vi "manual.vi"() -> ()   [LabVIEW 2010]
doc: "OCW v3.0\n\nCopyright 2008 by Will Grover\n\nhttp://wgrover.com\n\nPermission is hereby granted, free of charge, to any person obtaining a copy of this software and associated documentation files (the \"Software\"), to deal in the Software without restriction, including without limitation the rights to use, copy, modify, merge, publish, distribute, sublicense, and/or sell copies of the Software, and to permit persons to whom the Software is furnished to do so, subject to the following conditions:\n\nThe above copyright notice and this permission notice shall be included in all copies or substantial portions of the Software.\n\nTHE SOFTWARE IS PROVIDED \"AS IS\", WITHOUT WARRANTY OF ANY KIND, EXPRESS OR IMPLIED, INCLUDING BUT NOT LIMITED TO THE WARRANTIES OF MERCHANTABILITY, FITNESS FOR A PARTICULAR PURPOSE AND NONINFRINGEMENT. IN NO EVENT SHALL THE AUTHORS OR COPYRIGHT HOLDERS BE LIABLE FOR ANY CLAIM, DAMAGES OR OTHER LIABILITY, WHETHER IN AN ACTION OF CONTRACT, TORT OR OTHERWISE, ARISING FROM, OUT OF OR IN CONNECTION WITH THE SOFTWARE OR THE USE OR OTHER DEALINGS IN THE SOFTWARE."
panel:
  in  "HPLC valve setting":i32=1 min=1 max=2 step=1
  in  "Example button":bool
  out "ScanCode":i16=3
  in  "Valves":bool[](array[boolean])=[FALSE, FALSE, FALSE, FALSE, FALSE, FALSE, FALSE, FALSE, FALSE, FALSE, FALSE, FALSE, FALSE, FALSE, FALSE, FALSE]
  # "7"
  # "8"
  # "6"
  # "9"
  # "From\nwater"
  # "From\nmedia"
  # "From\ncells"
  # "to\nSMR"
  # "1"
  # "0"
  # "2"
  # "to\nSMR"
  # "From\ncells"
  # "From\nmedia"
  # "From\nwater"
  # "13"
  # "3"
  # "11"
  # "12"
  # "4"
  # "10"
  # "5"
  # "Make sure \"listener.vi\" is running before running this program.  This program controls the valves by (1) clicking on the above controls, (2) pressing the below keyboard shortcuts, and (3) pressing buttons like the one on the left.  This program can run while valve control programs (like OCW) are also running.  When adding additional keyboard controls, use the \"ScanCode\" output to determine the scan code returned by the key."
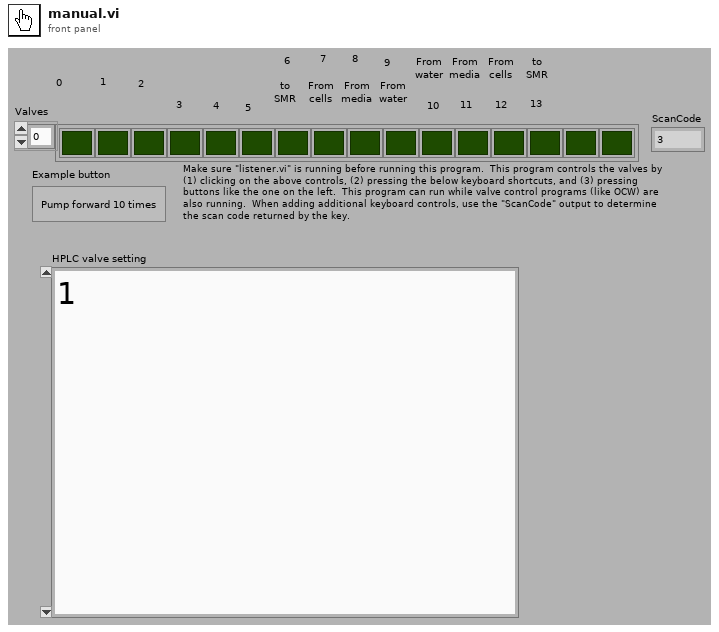
[diagram p1: front panel]
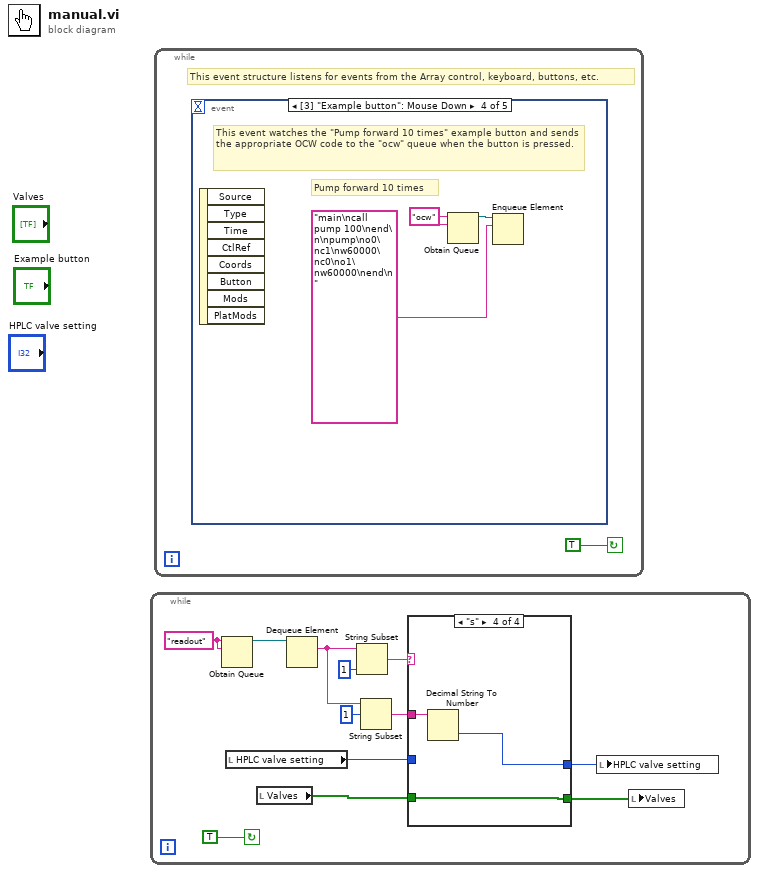
[diagram p0: block diagram]
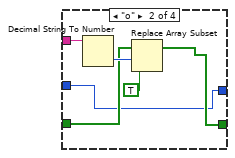
[diagram p3: hidden frame]
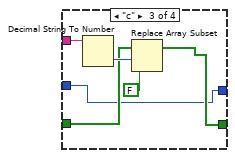
[diagram p4: hidden frame]
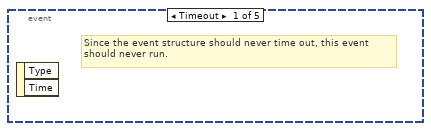
[diagram p5: hidden frame]
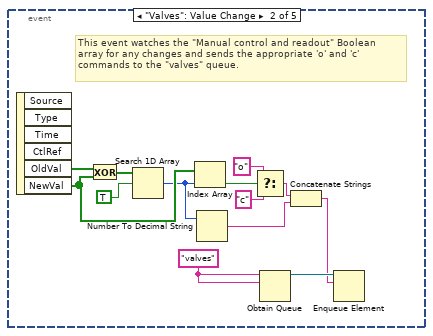
[diagram p6: hidden frame]
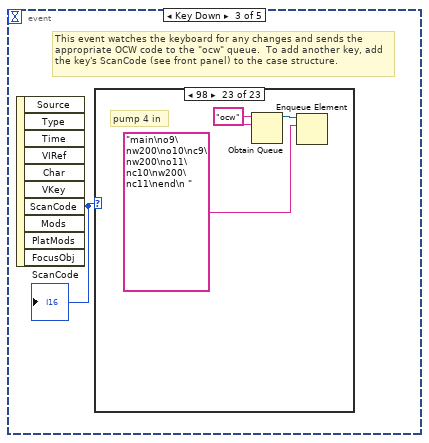
[diagram p7: hidden frame]
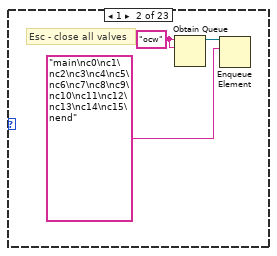
[diagram p9: hidden frame]
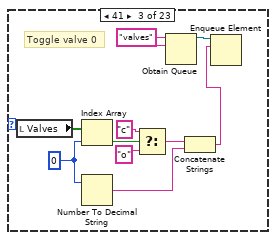
[diagram p10: hidden frame]
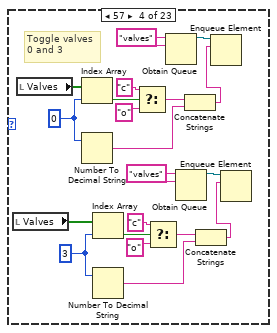
[diagram p11: hidden frame]
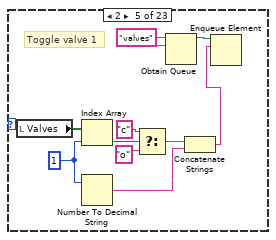
[diagram p12: hidden frame]
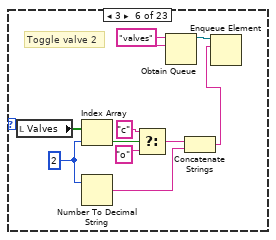
[diagram p13: hidden frame]
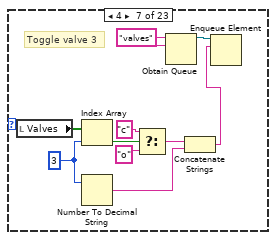
[diagram p14: hidden frame]
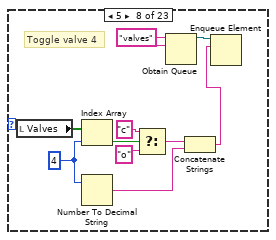
[diagram p15: hidden frame]
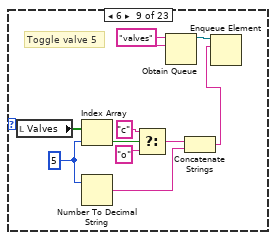
[diagram p16: hidden frame]
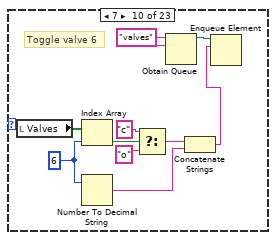
[diagram p17: hidden frame]
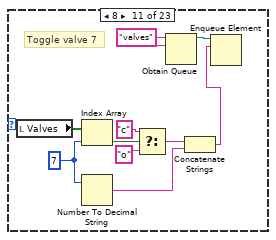
[diagram p18: hidden frame]
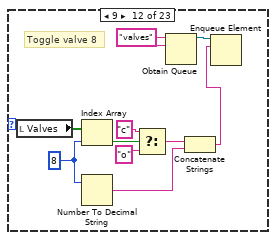
[diagram p19: hidden frame]
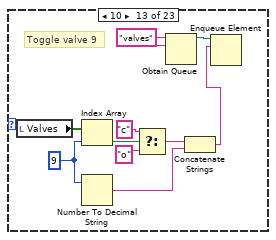
[diagram p20: hidden frame]
diagram:
  n1 = while {
    stop <- TRUE continue-if-true
    w11 = "readout" ("name (unnamed)")
    n2 = Obtain Queue(name (unnamed)=w11, element data type=w11) -> (queue out=w10:refnum<queue>)  [unwired: 3 in, 2 out]
    n3 = local read "HPLC valve setting"() -> (w2:i32)
    n4 = local read "Valves"() -> (w4:bool[])
    n5 = Dequeue Element(queue=w10) -> (element=w7:string)  [unwired: 1 in, 4 out]
    n6 = String Subset(string=w7, length (rest)=1 ("length (rest)")) -> (substring=w5:string)  [unwired: 1 out]
    n7 = String Subset(string=w7, offset (0)=1) -> (substring=w6:string)  [unwired: 1 out]
    n8 = case shown="\"s\"" w5 {
      tunnel: w6 -> [_ w20 w26 w29]
      tunnel: [w14 w17 w23 w28] -> w3
      tunnel: w4 -> [w14 w16 w22 w28]
      tunnel: w2 -> [w13 w15 w21 _]
      tunnel: [w13 w15 w21 w27] -> w1
      frame "", Default {
      }
      frame "o" {
        n9 = Decimal String To Number(string=w20) -> (number=w19:i32)  [unwired: 3 out]
        n10 = Replace Array Subset(array=w16, new element=TRUE, index=w19) -> (w17:bool[])
      }
      frame "c" {
        n11 = Decimal String To Number(string=w26) -> (number=w25:i32)  [unwired: 3 out]
        n12 = Replace Array Subset(array=w22, new element=FALSE, index=w25) -> (w23:bool[])
      }
      frame "s" {
        n13 = Decimal String To Number(string=w29) -> (number=w27:i32)  [unwired: 3 out]
      }
    }
    n14 = local write "HPLC valve setting"(w1) -> ()
    n15 = local write "Valves"(w3) -> ()
  }
  n16 = while {
    stop <- TRUE continue-if-true
    # "This event structure listens for events from the Array control, keyboard, buttons, etc."
    n17 = event shown="[3] \"Example button\": Mouse Down" {
      selector: _ -> [_ _ _ _ _]
      dyn-events: _ -> [_ _ _ _ _]
      timeout: _ -> [_ _ _ _ _]
      event Timeout {
        # "Since the event structure should never time out, this event should never run."
        n18 = event-data() -> ()  [unwired: 3 out]
      }
      event "Valves": Value Change {
        w42 = "valves" ("name (unnamed)")
        # "This event watches the \"Manual control and readout\" Boolean\narray for any changes and sends the appropriate 'o' and 'c'\ncommands to the \"valves\" queue."
        n19 = event-data() -> ("OldVal"=w41:bool[], "NewVal"=w38:bool[])  [unwired: 5 out]
        n20 = Exclusive Or(1:w38, 2:w41) -> (0:w40:bool[])
        n21 = Search 1D Array(1D array=w40, element=TRUE) -> (index of element=w34:i32)  [unwired: 1 out]
        n22 = Index Array(array=w38, index=w34) -> (element=w37:bool)
        n23 = Number To Decimal String(number=w34) -> (decimal integer string=w32:string)  [unwired: 1 out]
        n24 = Select(t="o", s=w37, f="c") -> (s? t:f=w33:string)
        n25 = Obtain Queue(name (unnamed)=w42, element data type=w42) -> (queue out=w43:refnum<queue>)  [unwired: 3 in, 2 out]
        n26 = Concatenate Strings(w33, w32) -> (w31:string)
        n27 = Enqueue Element(queue=w43, element=w31) -> ()  [unwired: 1 in, 4 out]
      }
      event Key Down {
        # "This event watches the keyboard for any changes and sends the appropriate OCW code to the \"ocw\" queue.  To add another key, add the key's ScanCode (see front panel) to the case structure."
        n28 = event-data() -> ("ScanCode"=w44:i16)  [unwired: 10 out]
        "ScanCode" <- w44
        n29 = case shown="98" w44 {
          frame 0, Default {
            # "The default case is empty so that nothing happens if non-monitored keys are pressed."
          }
          frame 1 {
            w47 = "ocw" ("name (unnamed)")
            # "Esc - close all valves"
            n30 = Obtain Queue(name (unnamed)=w47, element data type=w47) -> (queue out=w45:refnum<queue>)  [unwired: 3 in, 2 out]
            n31 = Enqueue Element(queue=w45, element="main\nc0\nc1\nc2\nc3\nc4\nc5\nc6\nc7\nc8\nc9\nc10\nc11\nc12\nc13\nc14\nc15\nend") -> ()  [unwired: 1 in, 4 out]
          }
          frame 41 {
            w51 = 0
            w56 = "valves" ("name (unnamed)")
            # "Toggle valve 0"
            n32 = local read "Valves"() -> (w55:bool[])
            n33 = Index Array(array=w55, index=w51) -> (element=w54:bool)
            n34 = Number To Decimal String(number=w51) -> (decimal integer string=w49:string)  [unwired: 1 out]
            n35 = Select(t="c", s=w54, f="o") -> (s? t:f=w50:string)
            n36 = Obtain Queue(name (unnamed)=w56, element data type=w56) -> (queue out=w57:refnum<queue>)  [unwired: 3 in, 2 out]
            n37 = Concatenate Strings(w50, w49) -> (w48:string)
            n38 = Enqueue Element(queue=w57, element=w48) -> ()  [unwired: 1 in, 4 out]
          }
          frame 57 {
            w63 = 3
            w59 = "valves" ("name (unnamed)")
            w71 = 0
            w76 = "valves" ("name (unnamed)")
            # "Toggle valves\n0 and 3"
            n39 = local read "Valves"() -> (w67:bool[])
            n40 = local read "Valves"() -> (w75:bool[])
            n41 = Index Array(array=w75, index=w71) -> (element=w74:bool)
            n42 = Number To Decimal String(number=w71) -> (decimal integer string=w69:string)  [unwired: 1 out]
            n43 = Index Array(array=w67, index=w63) -> (element=w60:bool)
            n44 = Number To Decimal String(number=w63) -> (decimal integer string=w65:string)  [unwired: 1 out]
            n45 = Select(t="c", s=w74, f="o") -> (s? t:f=w70:string)
            n46 = Select(t="c", s=w60, f="o") -> (s? t:f=w64:string)
            n47 = Obtain Queue(name (unnamed)=w76, element data type=w76) -> (queue out=w77:refnum<queue>)  [unwired: 3 in, 2 out]
            n48 = Obtain Queue(name (unnamed)=w59, element data type=w59) -> (queue out=w58:refnum<queue>)  [unwired: 3 in, 2 out]
            n49 = Concatenate Strings(w70, w69) -> (w68:string)
            n50 = Concatenate Strings(w64, w65) -> (w66:string)
            n51 = Enqueue Element(queue=w77, element=w68) -> ()  [unwired: 1 in, 4 out]
            n52 = Enqueue Element(queue=w58, element=w66) -> ()  [unwired: 1 in, 4 out]
          }
          frame 2 {
            w81 = 1
            w86 = "valves" ("name (unnamed)")
            # "Toggle valve 1"
            n53 = local read "Valves"() -> (w85:bool[])
            n54 = Index Array(array=w85, index=w81) -> (element=w84:bool)
            n55 = Number To Decimal String(number=w81) -> (decimal integer string=w79:string)  [unwired: 1 out]
            n56 = Select(t="c", s=w84, f="o") -> (s? t:f=w80:string)
            n57 = Obtain Queue(name (unnamed)=w86, element data type=w86) -> (queue out=w87:refnum<queue>)  [unwired: 3 in, 2 out]
            n58 = Concatenate Strings(w80, w79) -> (w78:string)
            n59 = Enqueue Element(queue=w87, element=w78) -> ()  [unwired: 1 in, 4 out]
          }
          frame 3 {
            w91 = 2
            w96 = "valves" ("name (unnamed)")
            # "Toggle valve 2"
            n60 = local read "Valves"() -> (w95:bool[])
            n61 = Index Array(array=w95, index=w91) -> (element=w94:bool)
            n62 = Number To Decimal String(number=w91) -> (decimal integer string=w89:string)  [unwired: 1 out]
            n63 = Select(t="c", s=w94, f="o") -> (s? t:f=w90:string)
            n64 = Obtain Queue(name (unnamed)=w96, element data type=w96) -> (queue out=w97:refnum<queue>)  [unwired: 3 in, 2 out]
            n65 = Concatenate Strings(w90, w89) -> (w88:string)
            n66 = Enqueue Element(queue=w97, element=w88) -> ()  [unwired: 1 in, 4 out]
          }
          frame 4 {
            w101 = 3
            w106 = "valves" ("name (unnamed)")
            # "Toggle valve 3"
            n67 = local read "Valves"() -> (w105:bool[])
            n68 = Index Array(array=w105, index=w101) -> (element=w104:bool)
            n69 = Number To Decimal String(number=w101) -> (decimal integer string=w99:string)  [unwired: 1 out]
            n70 = Select(t="c", s=w104, f="o") -> (s? t:f=w100:string)
            n71 = Obtain Queue(name (unnamed)=w106, element data type=w106) -> (queue out=w107:refnum<queue>)  [unwired: 3 in, 2 out]
            n72 = Concatenate Strings(w100, w99) -> (w98:string)
            n73 = Enqueue Element(queue=w107, element=w98) -> ()  [unwired: 1 in, 4 out]
          }
          frame 5 {
            w111 = 4
            w116 = "valves" ("name (unnamed)")
            # "Toggle valve 4"
            n74 = local read "Valves"() -> (w115:bool[])
            n75 = Index Array(array=w115, index=w111) -> (element=w114:bool)
            n76 = Number To Decimal String(number=w111) -> (decimal integer string=w109:string)  [unwired: 1 out]
            n77 = Select(t="c", s=w114, f="o") -> (s? t:f=w110:string)
            n78 = Obtain Queue(name (unnamed)=w116, element data type=w116) -> (queue out=w117:refnum<queue>)  [unwired: 3 in, 2 out]
            n79 = Concatenate Strings(w110, w109) -> (w108:string)
            n80 = Enqueue Element(queue=w117, element=w108) -> ()  [unwired: 1 in, 4 out]
          }
          frame 6 {
            w121 = 5
            w126 = "valves" ("name (unnamed)")
            # "Toggle valve 5"
            n81 = local read "Valves"() -> (w125:bool[])
            n82 = Index Array(array=w125, index=w121) -> (element=w124:bool)
            n83 = Number To Decimal String(number=w121) -> (decimal integer string=w119:string)  [unwired: 1 out]
            n84 = Select(t="c", s=w124, f="o") -> (s? t:f=w120:string)
            n85 = Obtain Queue(name (unnamed)=w126, element data type=w126) -> (queue out=w127:refnum<queue>)  [unwired: 3 in, 2 out]
            n86 = Concatenate Strings(w120, w119) -> (w118:string)
            n87 = Enqueue Element(queue=w127, element=w118) -> ()  [unwired: 1 in, 4 out]
          }
          frame 7 {
            w131 = 6
            w136 = "valves" ("name (unnamed)")
            # "Toggle valve 6"
            n88 = local read "Valves"() -> (w135:bool[])
            n89 = Index Array(array=w135, index=w131) -> (element=w134:bool)
            n90 = Number To Decimal String(number=w131) -> (decimal integer string=w129:string)  [unwired: 1 out]
            n91 = Select(t="c", s=w134, f="o") -> (s? t:f=w130:string)
            n92 = Obtain Queue(name (unnamed)=w136, element data type=w136) -> (queue out=w137:refnum<queue>)  [unwired: 3 in, 2 out]
            n93 = Concatenate Strings(w130, w129) -> (w128:string)
            n94 = Enqueue Element(queue=w137, element=w128) -> ()  [unwired: 1 in, 4 out]
          }
          frame 8 {
            w141 = 7
            w146 = "valves" ("name (unnamed)")
            # "Toggle valve 7"
            n95 = local read "Valves"() -> (w145:bool[])
            n96 = Index Array(array=w145, index=w141) -> (element=w144:bool)
            n97 = Number To Decimal String(number=w141) -> (decimal integer string=w139:string)  [unwired: 1 out]
            n98 = Select(t="c", s=w144, f="o") -> (s? t:f=w140:string)
            n99 = Obtain Queue(name (unnamed)=w146, element data type=w146) -> (queue out=w147:refnum<queue>)  [unwired: 3 in, 2 out]
            n100 = Concatenate Strings(w140, w139) -> (w138:string)
            n101 = Enqueue Element(queue=w147, element=w138) -> ()  [unwired: 1 in, 4 out]
          }
          frame 9 {
            w151 = 8
            w156 = "valves" ("name (unnamed)")
            # "Toggle valve 8"
            n102 = local read "Valves"() -> (w155:bool[])
            n103 = Index Array(array=w155, index=w151) -> (element=w154:bool)
            n104 = Number To Decimal String(number=w151) -> (decimal integer string=w149:string)  [unwired: 1 out]
            n105 = Select(t="c", s=w154, f="o") -> (s? t:f=w150:string)
            n106 = Obtain Queue(name (unnamed)=w156, element data type=w156) -> (queue out=w157:refnum<queue>)  [unwired: 3 in, 2 out]
            n107 = Concatenate Strings(w150, w149) -> (w148:string)
            n108 = Enqueue Element(queue=w157, element=w148) -> ()  [unwired: 1 in, 4 out]
          }
          frame 10 {
            w161 = 9
            w166 = "valves" ("name (unnamed)")
            # "Toggle valve 9"
            n109 = local read "Valves"() -> (w165:bool[])
            n110 = Index Array(array=w165, index=w161) -> (element=w164:bool)
            n111 = Number To Decimal String(number=w161) -> (decimal integer string=w159:string)  [unwired: 1 out]
            n112 = Select(t="c", s=w164, f="o") -> (s? t:f=w160:string)
            n113 = Obtain Queue(name (unnamed)=w166, element data type=w166) -> (queue out=w167:refnum<queue>)  [unwired: 3 in, 2 out]
            n114 = Concatenate Strings(w160, w159) -> (w158:string)
            n115 = Enqueue Element(queue=w167, element=w158) -> ()  [unwired: 1 in, 4 out]
          }
          frame 11 {
            w171 = 10
            w176 = "valves" ("name (unnamed)")
            # "Toggle valve 10"
            n116 = local read "Valves"() -> (w175:bool[])
            n117 = Index Array(array=w175, index=w171) -> (element=w174:bool)
            n118 = Number To Decimal String(number=w171) -> (decimal integer string=w169:string)  [unwired: 1 out]
            n119 = Select(t="c", s=w174, f="o") -> (s? t:f=w170:string)
            n120 = Obtain Queue(name (unnamed)=w176, element data type=w176) -> (queue out=w177:refnum<queue>)  [unwired: 3 in, 2 out]
            n121 = Concatenate Strings(w170, w169) -> (w168:string)
            n122 = Enqueue Element(queue=w177, element=w168) -> ()  [unwired: 1 in, 4 out]
          }
          frame 12 {
            w181 = 11
            w186 = "valves" ("name (unnamed)")
            # "Toggle valve 11"
            n123 = local read "Valves"() -> (w185:bool[])
            n124 = Index Array(array=w185, index=w181) -> (element=w184:bool)
            n125 = Number To Decimal String(number=w181) -> (decimal integer string=w179:string)  [unwired: 1 out]
            n126 = Select(t="c", s=w184, f="o") -> (s? t:f=w180:string)
            n127 = Obtain Queue(name (unnamed)=w186, element data type=w186) -> (queue out=w187:refnum<queue>)  [unwired: 3 in, 2 out]
            n128 = Concatenate Strings(w180, w179) -> (w178:string)
            n129 = Enqueue Element(queue=w187, element=w178) -> ()  [unwired: 1 in, 4 out]
          }
          frame 53 {
            w189 = "ocw" ("name (unnamed)")
            # "pump 2 out"
            n130 = Obtain Queue(name (unnamed)=w189, element data type=w189) -> (queue out=w190:refnum<queue>)  [unwired: 3 in, 2 out]
            n131 = Enqueue Element(queue=w190, element="main\no5\nw100\no4\nc5\nw100\no3\nc4\nw100\nc3\nend\n ") -> ()  [unwired: 1 in, 4 out]
          }
          frame 69 {
            w192 = "ocw" ("name (unnamed)")
            # "pump 1 out"
            n132 = Obtain Queue(name (unnamed)=w192, element data type=w192) -> (queue out=w193:refnum<queue>)  [unwired: 3 in, 2 out]
            n133 = Enqueue Element(queue=w193, element="main\no2\nw100\no1\nc2\nw100\no0\nc1\nw100\nc0\nend\n ") -> ()  [unwired: 1 in, 4 out]
          }
          frame 71 {
            w195 = "ocw" ("name (unnamed)")
            # "pump 1 in"
            n134 = Obtain Queue(name (unnamed)=w195, element data type=w195) -> (queue out=w196:refnum<queue>)  [unwired: 3 in, 2 out]
            n135 = Enqueue Element(queue=w196, element="main\no0\nw100\no1\nc0\nw100\no2\nc1\nw100\nc2\nend\n ") -> ()  [unwired: 1 in, 4 out]
          }
          frame 99 {
            w198 = "ocw" ("name (unnamed)")
            # "pump 2 in"
            n136 = Obtain Queue(name (unnamed)=w198, element data type=w198) -> (queue out=w199:refnum<queue>)  [unwired: 3 in, 2 out]
            n137 = Enqueue Element(queue=w199, element="main\no3\nw100\no4\nc3\nw100\no5\nc4\nw100\nc5\nend\n ") -> ()  [unwired: 1 in, 4 out]
          }
          frame 75 {
            w201 = "ocw" ("name (unnamed)")
            # "pump 3 out"
            n138 = Obtain Queue(name (unnamed)=w201, element data type=w201) -> (queue out=w202:refnum<queue>)  [unwired: 3 in, 2 out]
            n139 = Enqueue Element(queue=w202, element="main\no8\nw50\no7\nc8\nw50\no6\nc7\nw50\nc6\nend\n ") -> ()  [unwired: 1 in, 4 out]
          }
          frame 76 {
            w204 = "ocw" ("name (unnamed)")
            # "pump 4 out"
            n140 = Obtain Queue(name (unnamed)=w204, element data type=w204) -> (queue out=w205:refnum<queue>)  [unwired: 3 in, 2 out]
            n141 = Enqueue Element(queue=w205, element="main\no11\nw200\no10\nc11\nw200\no9\nc10\nw200\nc9\nend\n ") -> ()  [unwired: 1 in, 4 out]
          }
          frame 79 {
            w207 = "ocw" ("name (unnamed)")
            # "pump 3 in"
            n142 = Obtain Queue(name (unnamed)=w207, element data type=w207) -> (queue out=w208:refnum<queue>)  [unwired: 3 in, 2 out]
            n143 = Enqueue Element(queue=w208, element="main\no6\nw200\no7\nc6\nw200\no8\nc7\nw200\nc8\nend\n ") -> ()  [unwired: 1 in, 4 out]
          }
          frame 98 {
            w210 = "ocw" ("name (unnamed)")
            # "pump 4 in"
            n144 = Obtain Queue(name (unnamed)=w210, element data type=w210) -> (queue out=w211:refnum<queue>)  [unwired: 3 in, 2 out]
            n145 = Enqueue Element(queue=w211, element="main\no9\nw200\no10\nc9\nw200\no11\nc10\nw200\nc11\nend\n ") -> ()  [unwired: 1 in, 4 out]
          }
        }
      }
      event "Example button": Mouse Down {
        w213 = "ocw" ("name (unnamed)")
        # "This event watches the \"Pump forward 10 times\" example button and sends the appropriate OCW code to the \"ocw\" queue when the button is pressed."
        # "Pump forward 10 times"
        n146 = event-data() -> ()  [unwired: 9 out]
        n147 = Obtain Queue(name (unnamed)=w213, element data type=w213) -> (queue out=w214:refnum<queue>)  [unwired: 3 in, 2 out]
        n148 = Enqueue Element(queue=w214, element="main\ncall pump 100\nend\n\npump\no0\nc1\nw60000\nc0\no1\nw60000\nend\n ") -> ()  [unwired: 1 in, 4 out]
      }
      event "HPLC valve setting": Value Change {
        w219 = "valves" ("name (unnamed)")
        n149 = event-data() -> ("NewVal"=w218:i32)  [unwired: 6 out]
        n150 = Obtain Queue(name (unnamed)=w219, element data type=w219) -> (queue out=w220:refnum<queue>)  [unwired: 3 in, 2 out]
        n151 = Number To Decimal String(number=w218) -> (decimal integer string=w216:string)  [unwired: 1 out]
        n152 = Concatenate Strings("s", w216) -> (w215:string)
        n153 = Enqueue Element(queue=w220, element=w215) -> ()  [unwired: 1 in, 4 out]
      }
    }
  }
